vi "3D Array to RGBA.vi"(1 "3D Array":u8[][][](array[numeric])) -> (0 "RGBA":u32[][](array[numeric]))   [LabVIEW 2020, in "LV Tiff.lvlib"]
uses:
  LV Tiff.lvlib
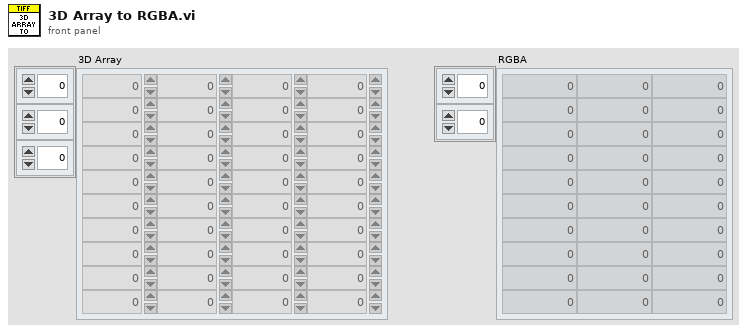
[diagram p1: front panel]
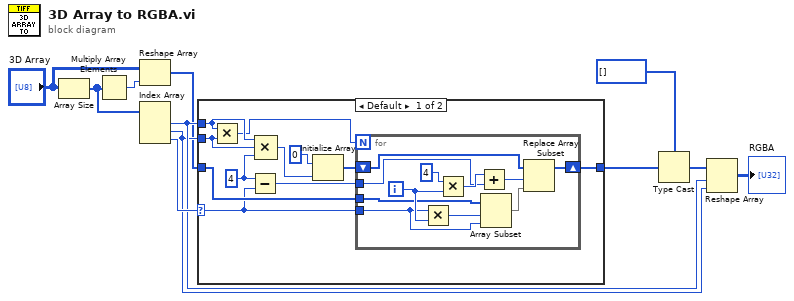
[diagram p0: block diagram]
diagram:
  n1 = Array Size(array="3D Array") -> (size(s)=w6:i32[])
  n2 = Multiply Array Elements(1:w6) -> (0:w5:i32)
  n3 = Reshape Array("3D Array", w5) -> (w4:u8[])
  n4 = Index Array(array=w6) -> (element #1=w8:i32, element #2=w7:i32, element #3=w11:i32)  [unwired: 3 in]
  n5 = case shown="Default" w11 {
    selector: w11 -> [w14 _]
    tunnel: w8 -> [w20 _]
    tunnel: w7 -> [w19 _]
    tunnel: w4 -> [w17 w34]
    tunnel: [w12 w34] -> w1
    frame Default {
      w15 = 4
      n6 = Multiply(x=w20, y=w19) -> (x*y=w18:i32)
      n7 = Subtract(x=w15, y=w14) -> (x-y=w13:i32)
      n8 = Compound Arithmetic op=MULTIPLY(w20, w19, w15) -> (w21:i32)
      n9 = Initialize Array(u8 0, w21) -> (w16:u8[])
      n10 = for {
        N: w18 -> [_]
        shift-right: [w27] -> w12
        shift-left: w16 -> [w33]
        tunnel: w17 -> [w30]
        tunnel: w14 -> [w28]
        tunnel: w13 -> [w24]
        i -> [w32]
        n11 = Multiply(x=w28, y=w32) -> (x*y=w29:i32)
        n12 = Multiply(x=4, y=w32) -> (x*y=w26:i32)
        n13 = Add(x=w26, y=w24) -> (x+y=w25:i32)
        n14 = Array Subset(array=w30, index=w29, length=w28) -> (w23:u8[])
        n15 = Replace Array Subset(array=w33, new element=w23, index=w25) -> (w27:u8[])
      }
    }
    frame 4 {
    }
  }
  n16 = Type Cast(type=u32[] [], x=w1) -> (*(type *) &x=w2:u32[])
  n17 = Reshape Array(w2, w8, w7) -> (→"RGBA":u32[][])
